vi "subVIweek7pt1.vi"(11 "AWG":dbl) -> (3 "Numeric":dbl)   [LabVIEW 2016]
uses:
  <vilib>/express/express arith-compare/Formula/XNode/ExpressFormulaBlockNode.xnode
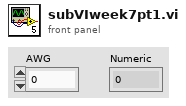
[diagram p1: front panel]
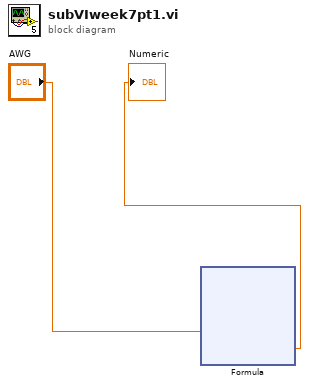
[diagram p0: block diagram]
diagram:
  n1 = xnode "Formula"("X1"="AWG") -> ("Result"=→"Numeric":dbl)  [unwired: 1 in, 1 out]
